vi "Setup TS.vi"(8 "error in":errorcluster, 11 "DeepU Test Stand in":refnum<class "DeepU Test Stand.lvclass">) -> (0 "error out":errorcluster, 3 "DeepU Test Stand out":refnum<class "DeepU Test Stand.lvclass">)   [LabVIEW 2019, in "Test Stands.lvlib" / "DeepU Test Stand.lvclass"]
uses:
  DeepU Test Stand.lvclass
  C:/Users/krio/Documents/LV_Projects/test-stand/App/Generic Test Stand/Generic Test Stand.lvclass
  DAC/DeepU/TC Temperature/DAC TC Temp DeepU.lvclass
  C:/Users/krio/Documents/LV_Projects/test-stand/App/DAC/DAC.lvclass
  DAC/DeepU/Keller Diff P 23X/DAC Keller Diff P 23X.lvclass
  DAC/DeepU/Keller BNC/DAC Keller BNC.lvclass
  DAC/DeepU/CS Humid/DAC CS Humid.lvclass
  DAC/DeepU/Inverter/DAC Inverter.lvclass
  DAC/DeepU/FTCU/DAC FTCU.lvclass
  DAC/DeepU/Jumo DP/DAC Jumo DP.lvclass
  DAC/DeepU/HS Vibration/DAC HS Vib.lvclass
  DAC/DAC.lvclass/DAC.ctl
  Generic Test Stand/Generic Test Stand.lvclass/Generic Test Stand.ctl
  DeepU Test Stand.lvclass/DeepU Test Stand.ctl
  Generic Test Stand/Generic Test Stand.lvclass
  DAC/DAC.lvclass
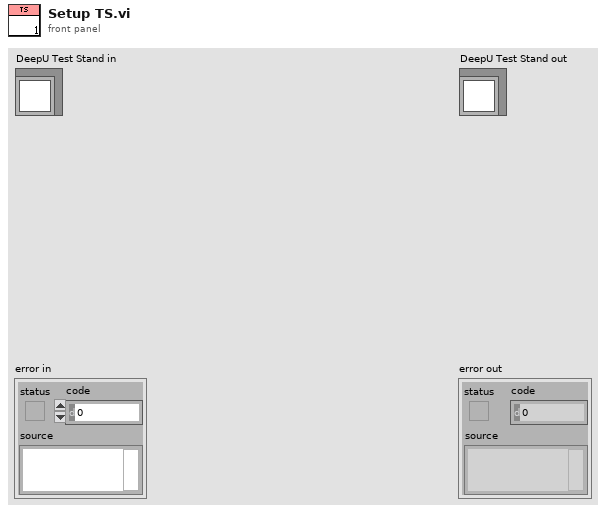
[diagram p1: front panel]
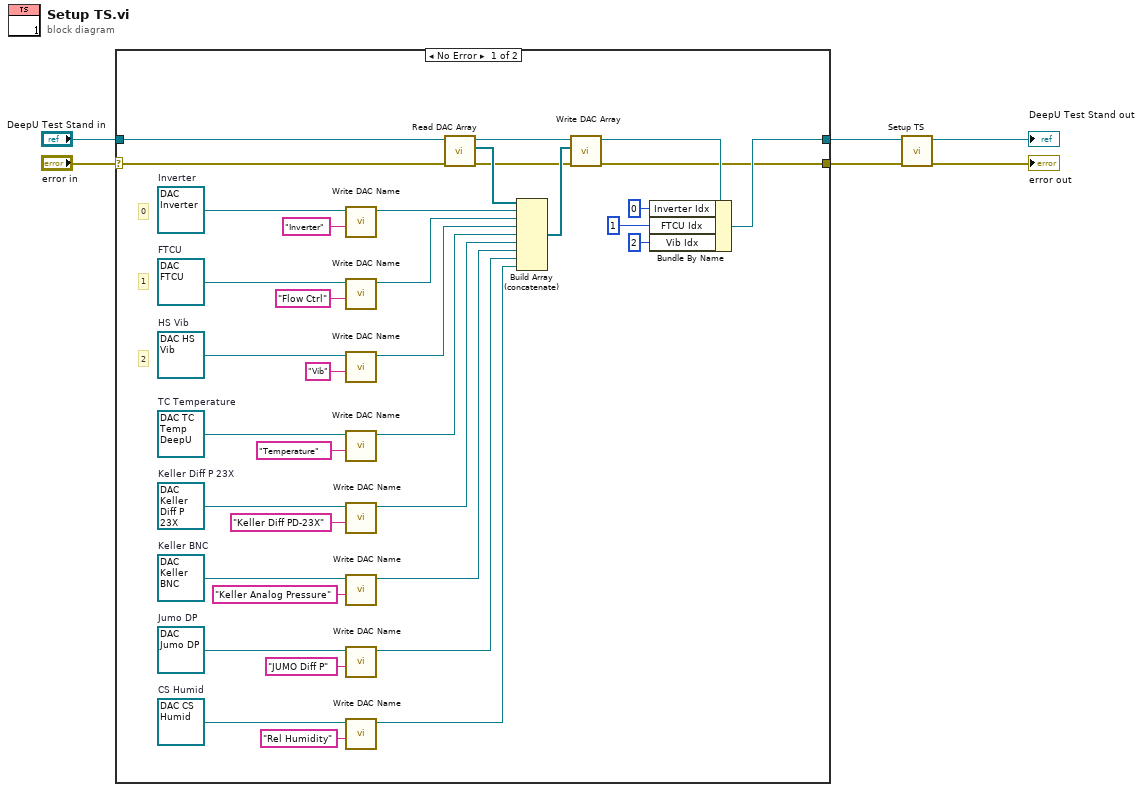
[diagram p0: block diagram]
diagram:
  n1 = case shown="No Error" "error in" {
    selector: "error in" -> [w21 w43]
    tunnel: "DeepU Test Stand in" -> [w42 w44]
    tunnel: [w19 w44] -> w2
    tunnel: [w16 w43] -> w1
    frame No Error {
      w9 = refnum<class "DAC HS Vib.lvclass"> refnum  # HS Vib
      w13 = refnum<class "DAC Jumo DP.lvclass"> refnum  # Jumo DP
      w15 = refnum<class "DAC FTCU.lvclass"> refnum  # FTCU
      w26 = refnum<class "DAC Inverter.lvclass"> refnum  # Inverter
      w30 = refnum<class "DAC CS Humid.lvclass"> refnum  # CS Humid
      w32 = refnum<class "DAC Keller BNC.lvclass"> refnum  # Keller BNC
      w34 = refnum<class "DAC Keller Diff P 23X.lvclass"> refnum  # Keller Diff P 23X
      w36 = refnum<class "DAC TC Temp DeepU.lvclass"> refnum  # TC Temperature
      # "2"
      # "1"
      # "0"
      n2 = call "Write DAC Name.vi"("DAC Name"="Inverter", "DAC in"=w26) -> ("DAC out"=w25:refnum<class "DAC Inverter.lvclass">)  [unwired: 8 in, 1 out]
      n3 = call "Write DAC Name.vi"("DAC Name"="Flow Ctrl", "DAC in"=w15) -> ("DAC out"=w24:refnum<class "DAC FTCU.lvclass">)  [unwired: 8 in, 1 out]
      n4 = call "Write DAC Name.vi"("DAC Name"="Vib", "DAC in"=w9) -> ("DAC out"=w8:refnum<class "DAC HS Vib.lvclass">)  [unwired: 8 in, 1 out]
      n5 = call "Write DAC Name.vi"("DAC Name"="Temperature", "DAC in"=w36) -> ("DAC out"=w27:refnum<class "DAC TC Temp DeepU.lvclass">)  [unwired: 8 in, 1 out]
      n6 = call "Write DAC Name.vi"("DAC Name"="Keller Diff PD-23X", "DAC in"=w34) -> ("DAC out"=w28:refnum<class "DAC Keller Diff P 23X.lvclass">)  [unwired: 8 in, 1 out]
      n7 = call "Write DAC Name.vi"("DAC Name"="Keller Analog Pressure", "DAC in"=w32) -> ("DAC out"=w29:refnum<class "DAC Keller BNC.lvclass">)  [unwired: 8 in, 1 out]
      n8 = call "Write DAC Name.vi"("DAC Name"="JUMO Diff P", "DAC in"=w13) -> ("DAC out"=w12:refnum<class "DAC Jumo DP.lvclass">)  [unwired: 8 in, 1 out]
      n9 = call "Write DAC Name.vi"("DAC Name"="Rel Humidity", "DAC in"=w30) -> ("DAC out"=w11:refnum<class "DAC CS Humid.lvclass">)  [unwired: 8 in, 1 out]
      n10 = call "Read DAC Array.vi"("error in (no error)"=w21, "Generic Test Stand in"=w42) -> ("error out"=w20:errorcluster, "DAC Array"=w41:refnum<class "DAC.lvclass">[], "Generic Test Stand out"=w40:refnum<class "DeepU Test Stand.lvclass">)  [unwired: 7 in]
      n11 = Build Array (concatenate)(w41, w25, w24, w8, w27, w28, w29, w12, w11) -> (w39:refnum<class "DAC.lvclass">[])
      n12 = call "Write DAC Array.vi"("error in (no error)"=w20, "DAC Array"=w39, "Generic Test Stand in"=w40) -> ("error out"=w16:errorcluster, "Generic Test Stand out"=w37:refnum<class "DeepU Test Stand.lvclass">)  [unwired: 7 in]
      n13 = Bundle By Name(cluster=w37, "Inverter Idx"=0 ("Inverter No"), "FTCU Idx"=1 ("FTCU No"), "Vib Idx"=2) -> (w19:refnum<class "DeepU Test Stand.lvclass">)
    }
    frame Error {
    }
  }
  n14 = call-parent "Setup TS.vi"("error in (no error)"=w1, "Generic Test Stand in"=w2) -> ("error out"=→"error out":errorcluster, "Generic Test Stand out"=→"DeepU Test Stand out":refnum<class "DeepU Test Stand.lvclass">)  [unwired: 8 in]
